vi "Dynamic Event Generation.vi"() -> ()   [LabVIEW 2023]
doc: "Demonstrates dynamic events. In this example, the Mouse Move event is not registered until the user clicks down on the card. The Mouse Move event is then unregistered on the Mouse Up event or when the user releases the mouse button. Dynamic Events gives the programmer control over when the events are registered."
panel:
  out "Picture":picture
  in  "Stop":bool
  out "Iteration Count":i32
  # "Overview: Demonstrates the use of the Register for Events function to dynamically register and unregister for events while a VI runs.\nInstructions:\n1. Run the VI.\n2. Click and drag the Picture. Note that the picture moves with the mouse, and the Iteration Count value increases, which shows that the Mouse Move event is firing.\n3. Drag the Picture to the lower area of the panel and stop dragging. Note that the Iteration Count value no longer changes, since the Mouse Move event was unregistered when the dragging stopped.\n4. Click Stop to stop the VI."
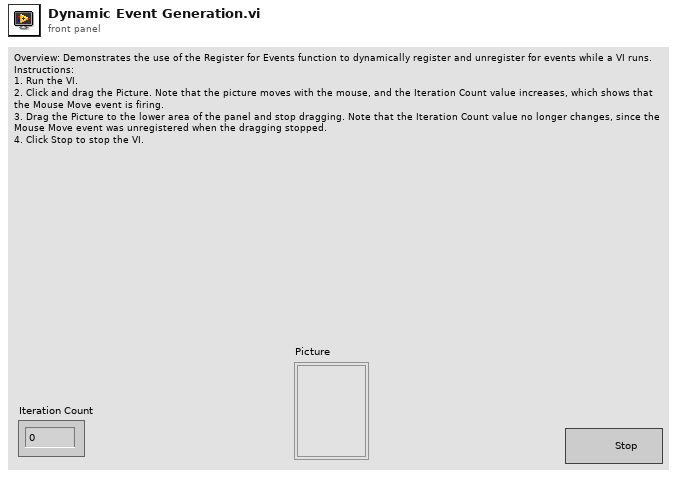
[diagram p1: front panel]
types:
  T1 = typedef "LVPoint32TypeDef.ctl" = cluster{"Horizontal":i32, "Vertical":i32}
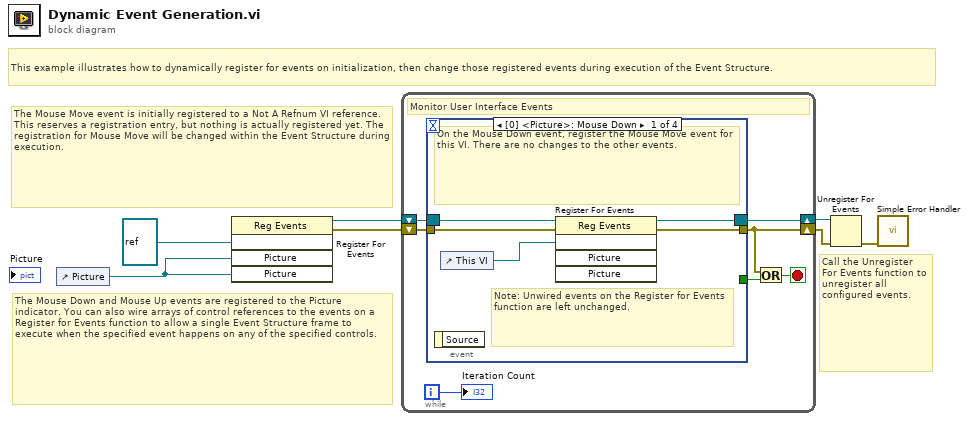
[diagram p0: block diagram]
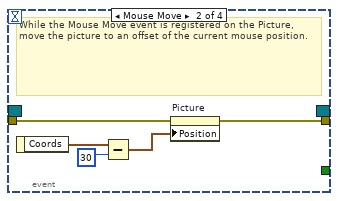
[diagram p2: hidden frame]
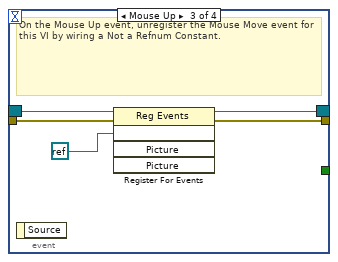
[diagram p3: hidden frame]
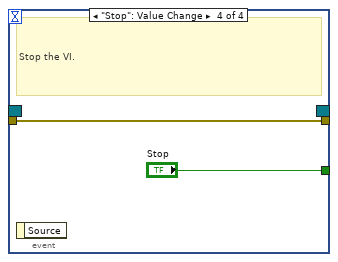
[diagram p4: hidden frame]
diagram:
  # "This example illustrates how to dynamically register for events on initialization, then change those registered events during execution of the Event Structure."
  # "Call the Unregister For Events function to unregister all configured events."
  # "The Mouse Move event is initially registered to a Not A Refnum VI reference. This reserves a registration entry, but nothing is actually registered yet. The registration for Mouse Move will be changed within the Event Structure during execution."
  # "The Mouse Down and Mouse Up events are registered to the Picture indicator. You can also wire arrays of control references to the events on a Register for Events function to allow a single Event Structure frame to execute when the specified event happens on any of the specified controls."
  n1 = control-ref of="Picture"() -> (w1:refnum<vi>)
  n2 = register-events(refnum<vi> refnum, w1, w1) -> (reference out=w7:refnum<event-registration>, error out=w4:errorcluster)  [unwired: 2 in]
  n3 = while {
    shift-right: [w12] -> w6
    shift-left: w7 -> [w13]
    shift-right: [w8] -> w3
    shift-left: w4 -> [w11]
    i -> [w14]
    stop <- w10 stop-if-true
    # "Monitor User Interface Events"
    n4 = event shown="[0] <Picture>: Mouse Down" {
      selector: w13 -> [w19 _ w29 _]
      dyn-events: [w18 _ w27 _] -> w12
      timeout: _ -> [_ _ _ _]
      tunnel: [_ _ _ "Stop"] -> w9
      tunnel: w11 -> [w17 w21 w26 w30]
      tunnel: [w16 w20 w25 w30] -> w8
      event Mouse Down {
        # "Note: Unwired events on the Register for Events function are left unchanged."
        # "On the Mouse Down event, register the Mouse Move event for this VI. There are no changes to the other events."
        n5 = event-data() -> ()  [unwired: 1 in, 1 out]
        n6 = control-ref of="This VI"() -> (w15:refnum<vi>)
        n7 = register-events(reference=w19, error in=w17, w15) -> (reference out=w18:refnum<event-registration>, error out=w16:errorcluster)  [unwired: 2 in]
      }
      event Mouse Move {
        # "While the Mouse Move event is registered on the Picture,  move the picture to an offset of the current mouse position."
        n8 = event-data() -> ("Coords"=w24:T1)  [unwired: 1 in]
        n9 = Subtract(x=w24, y=30) -> (x-y=w22:T1)
        n10 = property on="Picture" class="Pict"(error in=w21, "Position"=w22) -> (error out=w20:errorcluster)  [unwired: 1 in, 1 out]
      }
      event Mouse Up {
        # "On the Mouse Up event, unregister the Mouse Move event for this VI by wiring a Not a Refnum Constant."
        n11 = event-data() -> ()  [unwired: 1 in, 1 out]
        n12 = register-events(reference=w29, error in=w26, refnum<k0> refnum) -> (reference out=w27:refnum<event-registration>, error out=w25:errorcluster)  [unwired: 2 in]
      }
      event "Stop": Value Change {
        # "Stop the VI."
        n13 = event-data() -> ()  [unwired: 1 in, 1 out]
      }
    }
    n14 = Or(x=w8, y=w9) -> (x .or. y?=w10:bool)
    "Iteration Count" <- w14
  }
  n15 = Unregister For Events(event registration refnum=w6, error in=w3) -> (error out=w2:errorcluster)
  n16 = call <vilib>:"Simple Error Handler.vi"("error in (no error)"=w2) -> ()  [unwired: 4 in, 5 out]
